vi "STFT Spectrogram PtByPt.vi"(2 "window selector":i32(ring) items=["Hanning", "Hamming", "Blackman", "Exact Blackman", "Blackman-Harris"], 3 "initialize":bool, 4 "window length":i32=50, 5 "time increment":i32=1, 6 "sample length":i32=100, 7 "x":dbl format="%0.2f") -> (0 "error":i32, 1 "STFT Spectrogram {X}":dbl[][](array[numeric]))   [LabVIEW 2020, in "NI_PtbyPt.lvlib"]
doc: "Computes the signal energy distribution in the joint time-frequency domain using the short-time Fourier transform (STFT) algorithm."
uses:
  NI_PtbyPt.lvlib
  Hanning Window (DBL).vi
  Hamming Window (DBL).vi
  Blackman Window (DBL).vi
  Exact Blackman Window (DBL).vi
  Blackman-Harris Window (DBL).vi
  Unit Vector (DBL).vi
  AllCosWindow (DBL).vi
  NI_AALBase.lvlib
  NI_AALPro.lvlib
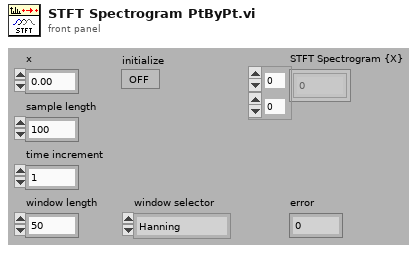
[diagram p1: front panel]
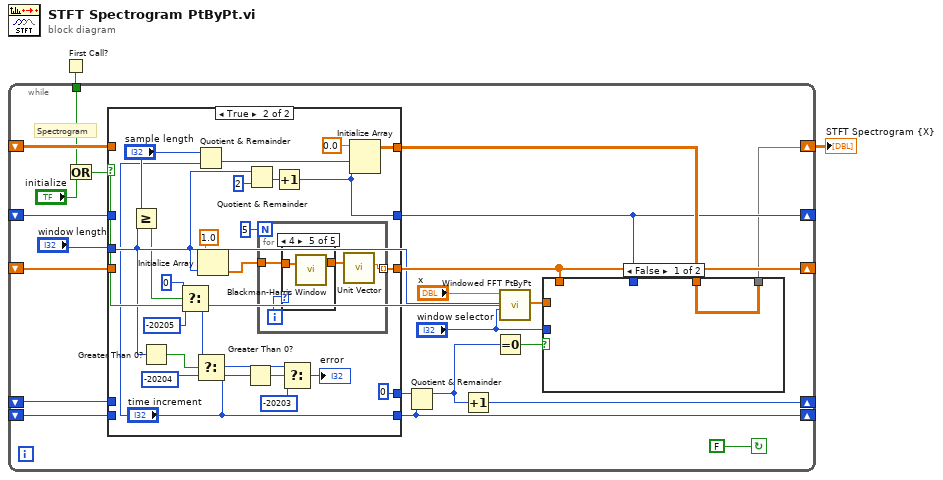
[diagram p0: block diagram]
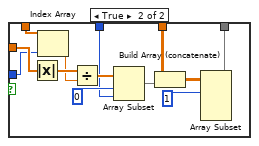
[diagram p2: hidden frame]
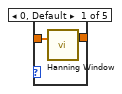
[diagram p4: hidden frame]
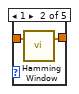
[diagram p5: hidden frame]
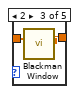
[diagram p6: hidden frame]
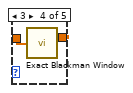
[diagram p7: hidden frame]
diagram:
  n1 = First Call?() -> (First Call?: T/F=w2:bool)
  n2 = while {
    tunnel: w2 -> [w5]
    shift-left: _ -> [w22]
    shift-right: [w9] -> _
    shift-left: _ -> [w23]
    shift-right: [w12] -> _
    shift-left: _ -> [w19]
    shift-right: [w16] -> _
    shift-left: _ -> [w18]
    shift-right: [w13] -> _
    shift-left: _ -> [w24]
    shift-right: [w4] -> w1
    stop <- FALSE continue-if-true
    # "Spectrogram"
    n3 = Or(x=w5, y="initialize") -> (x .or. y?=w6:bool)
    n4 = case shown="True" w6 {
      tunnel: [w42 w60] -> w20
      tunnel: [w39 0] -> w17
      tunnel: w19 -> [w43 _]
      tunnel: w24 -> [w42 _]
      tunnel: [w43 "time increment"] -> w16
      tunnel: [w41 w57] -> w12
      tunnel: [w40 w62] -> w9
      tunnel: w18 -> [w39 _]
      tunnel: w23 -> [w41 _]
      tunnel: w22 -> [w40 _]
      tunnel: "window length" -> [_ w51]
      frame False {
      }
      frame True {
        n5 = Greater Or Equal?(x="sample length", y=w51) -> (x >= y?=w49:bool)
        n6 = Greater Than 0?(x=w51) -> (x > 0?=w50:bool)
        n7 = Select(t=0, s=w49, f=-20205) -> (s? t:f=w47:i32)
        n8 = Quotient & Remainder(x="sample length", y="time increment") -> (floor(x/y)=w56:i32)  [unwired: 1 out]
        n9 = Select(t=w47, s=w50, f=-20204) -> (s? t:f=w54:i32)
        n10 = Initialize Array(1.0, w51) -> (w58:dbl[])
        n11 = Greater Than 0?(x="time increment") -> (x > 0?=w55:bool)
        n12 = Quotient & Remainder(x=w51, y=2) -> (floor(x/y)=w64:i32)  [unwired: 1 out]
        n13 = for {
          N: 5 -> [_]
          tunnel: w58 -> [w70]
          tunnel: [w68] -> w57 mode=indexing
          i -> [w71]
          n14 = case shown="4" w71 {
            tunnel: w70 -> [w73 w75 w77 w79 w81]
            tunnel: [w72 w74 w76 w78 w80] -> w69
            frame 0, Default {
              n15 = call-poly "Hanning Window.vi"("X"=w73) -> ("Windowed X"=w72:dbl[])  [unwired: 1 out]
            }
            frame 1 {
              n16 = call-poly "Hamming Window.vi"("X"=w75) -> ("Windowed X"=w74:dbl[])  [unwired: 1 out]
            }
            frame 2 {
              n17 = call-poly "Blackman Window.vi"("X"=w77) -> ("Windowed X"=w76:dbl[])  [unwired: 1 out]
            }
            frame 3 {
              n18 = call-poly "Exact Blackman Window.vi"("X"=w79) -> ("Windowed X"=w78:dbl[])  [unwired: 1 out]
            }
            frame 4 {
              n19 = call-poly "Blackman-Harris Window.vi"("X"=w81) -> ("Windowed X"=w80:dbl[])  [unwired: 1 out]
            }
          }
          n20 = call-poly "Unit Vector.vi"("Input Vector"=w69) -> ("norm"=w68:dbl)  [unwired: 8 in, 2 out]
        }
        n21 = Increment(x=w64) -> (x+1=w62:i32)
        n22 = Select(t=w54, s=w55, f=-20203) -> (s? t:f=→"error":i32)
        n23 = Initialize Array(0.0, w56, w62) -> (w60:dbl[][])
      }
    }
    n24 = Quotient & Remainder(x=w17, y=w16) -> (x-y*floor(x/y)=w15:i32)  [unwired: 1 out]
    n25 = Increment(x=w15) -> (x+1=w13:i32)
    n26 = Equal To 0?(x=w15) -> (x = 0?=w14:bool)
    n27 = call "Windowed FFT PtByPt.vi"("x"="x", "sample length"="window length", "window selector"="window selector", "initialize"=w6) -> ("Windowed FFT"=w21:cdb[])  [unwired: 1 in, 1 out]
    n28 = case shown="False" w14 {
      tunnel: w21 -> [_ w32]
      tunnel: w20 -> [w25 w30]
      tunnel: [w25 w33] -> w4
      tunnel: w12 -> [_ w29]
      tunnel: "window selector" -> [_ w28]
      tunnel: w9 -> [_ w27]
      frame False {
      }
      frame True {
        n29 = Absolute Value(x=w32) -> (abs(x)=w38:dbl[])
        n30 = Index Array(array=w29, index=w28) -> (element=w26:dbl)
        n31 = Divide(x=w38, y=w26) -> (x/y=w31:dbl[])
        n32 = Array Subset(array=w31, index=0 ("Array Index"), length=w27) -> (w36:dbl[])
        n33 = Build Array (concatenate)(w30, w36) -> (w35:dbl[][])
        n34 = Array Subset(array=w35, index (row)=1 ("Array Index")) -> (w33:dbl[][])  [unwired: 3 in]
      }
    }
  }
  "STFT Spectrogram {X}" <- w1
